vi "dump_photon_stream.vi"(5 "acq_mode":T1=2 items=["T2"=2, "T3"=3], 7 "sync":u64[](array[numeric]), 8 "error in (no error)":errorcluster, 9 "channels":u8[](array[numeric]), 10 "photon_records":u64[](array[numeric]), 11 "pcfs_hdf5_log in":refnum<class "pcfs_hdf5_log.lvclass">) -> (0 "error out":errorcluster, 3 "pcfs_hdf5_log out":refnum<class "pcfs_hdf5_log.lvclass">)   [LabVIEW 2015, in "pcfs_hdf5_log.lvclass"]
uses:
  pcfs_hdf5_log.lvclass
  lvoop_dll-master/picoquant_Tmodes.ctl
  pcfs_hdf5_log.lvclass/pcfs_hdf5_log.ctl
  <vilib>/UPVI/lvhdf5/dataset.llb/Append Element(s) to Dataset (Variant).vi
  <vilib>/UPVI/lvhdf5/dataset.llb/Append Element(s) to Dataset.xnode
  <vilib>/UPVI/lvhdf5/library.llb/HDF5 Ref.ctl
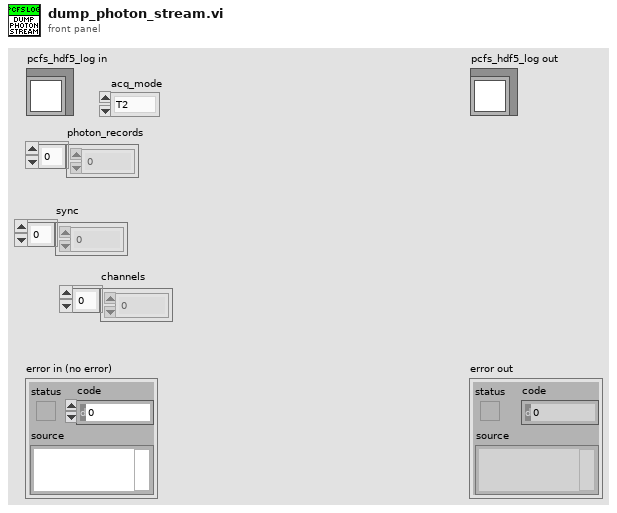
[diagram p1: front panel]
types:
  T1 = typedef "picoquant_Tmodes.ctl" = u16
  T2 = typedef "HDF5 Ref.ctl" = refnum<k1>
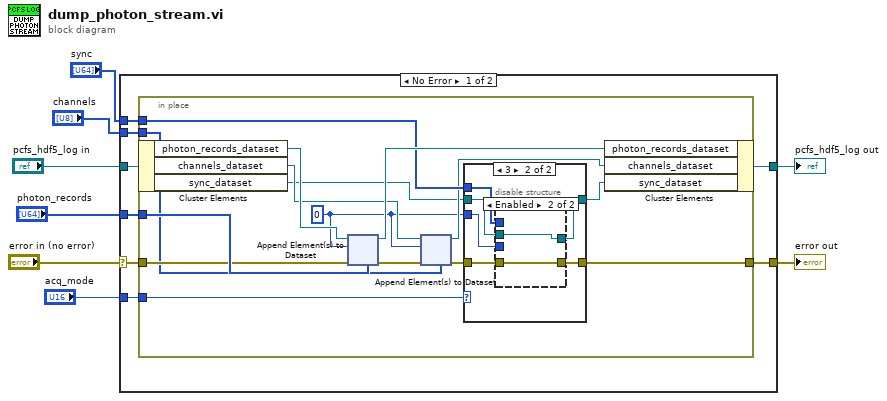
[diagram p0: block diagram]
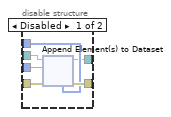
[diagram p3: hidden frame]
diagram:
  n1 = case shown="No Error" "error in (no error)" {
    selector: "error in (no error)" -> [w14 w73]
    tunnel: "pcfs_hdf5_log in" -> [w16 w72]
    tunnel: "photon_records" -> [w15 _]
    tunnel: [w13 w73] -> w5
    tunnel: "channels" -> [w12 _]
    tunnel: "sync" -> [w11 _]
    tunnel: "acq_mode" -> [w10 _]
    tunnel: [w9 w72] -> w1
    frame No Error {
      n2 = in-place {
        in-place-border: w15 -> [w29]
        in-place-border: w14 -> [w26]
        in-place-border: [w25] -> w13
        in-place-border: w12 -> [w24]
        in-place-border: w11 -> [w23]
        in-place-border: w10 -> [w22]
        w17 = 0 ("Dimension to Extend (0)")
        n3 = in-place-cluster #1(w16) -> ("photon_records_dataset"=w31:T2, "channels_dataset"=w21:T2, "sync_dataset"=w19:T2)
        n4 = xnode "Append Element(s) to Dataset"("Dimension to Extend (0)"=w17, "HDF5 Dataset Ref"=w31, "error in (no error)"=w26, "Data Element(s)"=w29) -> ("HDF5 Dataset out"=w30:T2, "error out"=w28:errorcluster)  [unwired: 2 out]
        n5 = xnode "Append Element(s) to Dataset"("Dimension to Extend (0)"=w17, "HDF5 Dataset Ref"=w21, "error in (no error)"=w28, "Data Element(s)"=w24) -> ("HDF5 Dataset out"=w20:T2, "error out"=w27:errorcluster)  [unwired: 2 out]
        n6 = case shown="3" w22 {
          tunnel: w27 -> [w33 w39]
          tunnel: [w33 w38] -> w25
          tunnel: w23 -> [_ w37]
          tunnel: w19 -> [w32 w36]
          tunnel: [w32 w35] -> w18
          tunnel: w17 -> [_ w34]
          frame 2, Default {
          }
          frame 3 {
            n7 = disable-structure shown="Enabled" {
              disable-tunnel: w39 -> [w45 w55]
              disable-tunnel: [w44 w55] -> w38
              disable-tunnel: w37 -> [w43 _]
              disable-tunnel: w36 -> [w42 w54]
              disable-tunnel: [w41 w54] -> w35
              disable-tunnel: w34 -> [w40 _]
              frame Disabled {
                n8 = xnode "Append Element(s) to Dataset"("Dimension to Extend (0)"=w40, "HDF5 Dataset Ref"=w42, "error in (no error)"=w45, "Data Element(s)"=w43) -> ("HDF5 Dataset out"=w41:T2, "error out"=w44:errorcluster)  [unwired: 2 out]
              }
              frame Enabled {
              }
            }
          }
        }
        n9 = in-place-cluster #1("photon_records_dataset"=w30, "channels_dataset"=w20, "sync_dataset"=w18) -> (w9:refnum<class "pcfs_hdf5_log.lvclass">)
      }
    }
    frame Error {
    }
  }
  "error out" <- w5
  "pcfs_hdf5_log out" <- w1
